vi "macro_vecBuilder3x1FIll.vi"   [LabVIEW 2019, in "Trajectory_Library.lvlib"]
uses:
  MatBuilder_Create.vi
  Trajectory_Library.lvlib
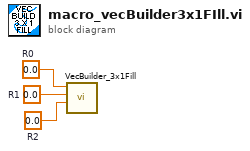
[diagram p0: block diagram]
diagram:
  w1 = 0.0  # R2
  w2 = 0.0  # R1
  w3 = 0.0  # R0
  n1 = call "VecBuilder_3x1Fill.vi"("R2"=w1, "R1"=w2, "R0"=w3) -> ()  [unwired: 8 in, 1 out]
